vi "InsertIntoShortcutMenu.vi"(8 "error in":errorcluster, 9 "menu ref in":refnum<k9>, 11 "node in":refnum<class "cRIO  node root.lvclass">) -> (0 "error out":errorcluster, 1 "menu ref out":refnum<k9>, 3 "node out":refnum<class "cRIO  node root.lvclass">)   [LabVIEW 2014, in "cRIO  node root.lvclass"]
doc: "Allows children to insert menu items without overriding ShortcutMenu.vi entirely. By default, called before Add/Remove."
uses:
  cRIO  node root.lvclass
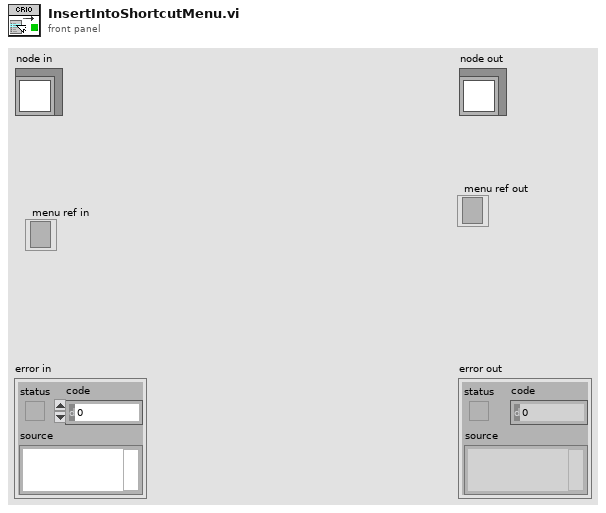
[diagram p1: front panel]
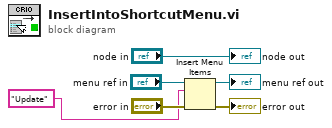
[diagram p0: block diagram]
diagram:
  n1 = Insert Menu Items(6:"error in", 8:"Update", 9:"menu ref in") -> (0:→"error out":errorcluster, 3:→"menu ref out":refnum<k9>)  [unwired: 3 in, 1 out]
  "node out" <- "node in"
